vi "test_ccd_OpenAndClose.vi"(8 "error in":errorcluster, 11 "CCD in":refnum<class "CCD.lvclass">) -> (0 "error out":errorcluster, 3 "CCD out":refnum<class "CCD.lvclass">)   [LabVIEW 2020, in "horiba.test.lvlib"]
uses:
  horiba.test.lvlib
  <vilib>/addons/_JKI Toolkits/Caraya/classes/Assert/Assert True.vi
  <vilib>/addons/_JKI Toolkits/Caraya/classes/Assert/Assert False.vi
  Classes/CCD/CCD.lvclass
panel:
  # "Connector Pane"
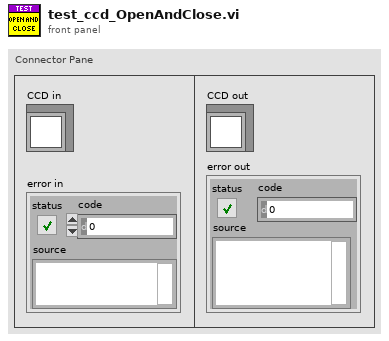
[diagram p1: front panel]
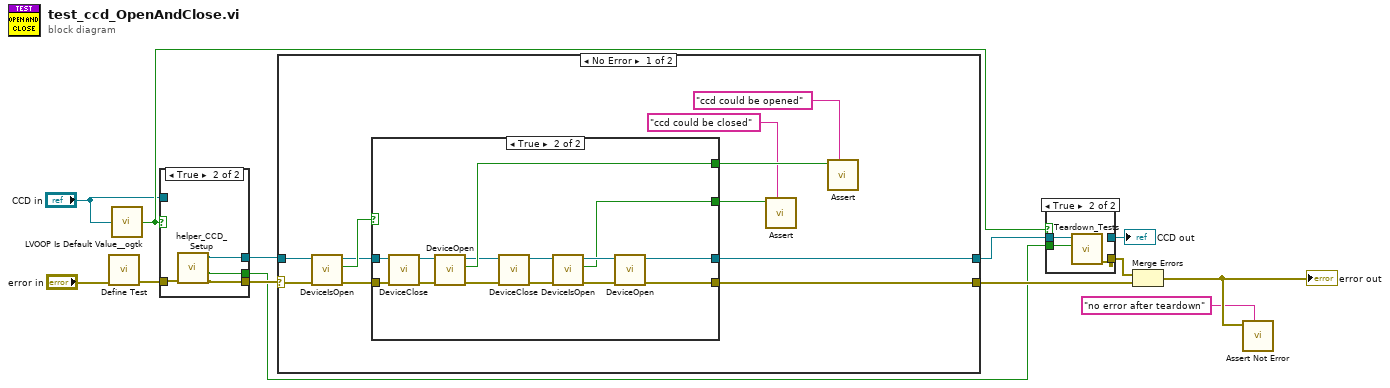
[diagram p0: block diagram]
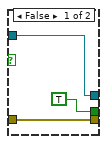
[diagram p3: hidden frame]
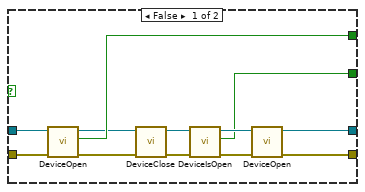
[diagram p4: hidden frame]
diagram:
  n1 = call <vilib>:"Define Test.vi"("error in (no error)"="error in") -> ("error out"=w9:errorcluster)  [unwired: 9 in, 1 out]
  n2 = call <userlib>:"LVOOP Is Default Value__ogtk.vi"("Object"="CCD in") -> ("Is Default Value?"=w3:bool)
  n3 = case shown="True" w3 {
    tunnel: w9 -> [w16 w17]
    tunnel: [w16 w19] -> w8
    tunnel: [w14 w20] -> w7
    tunnel: [TRUE ("Module Was Already Running?") w18] -> w4
    tunnel: "CCD in" -> [w14 _]
    frame False {
    }
    frame True {
      n4 = call "helper_CCD_Setup.vi"("error in"=w17) -> ("error out"=w19:errorcluster, "Module Was Already Running?"=w18:bool, "CCD out"=w20:refnum<class "CCD.lvclass">)  [unwired: 7 in, 1 out]
    }
  }
  n5 = case shown="No Error" w8 {
    selector: w8 -> [w30 w59]
    tunnel: [w21 w58] -> w12
    tunnel: w7 -> [w31 w58]
    tunnel: [w22 w59] -> w11
    frame No Error {
      n6 = call-dynamic "DeviceIsOpen.vi"("error in (no error)"=w30, "CCD in"=w31) -> ("error out"=w27:errorcluster, "device is open?"=w29:bool, "CCD out"=w28:refnum<class "CCD.lvclass">)  [unwired: 6 in, 1 out]
      n7 = case shown="True" w29 {
        tunnel: w28 -> [w42 w47]
        tunnel: w27 -> [w43 w48]
        tunnel: [w41 w57] -> w26
        tunnel: [w32 w44] -> w23
        tunnel: [w34 w50] -> w22
        tunnel: [w33 w49] -> w21
        frame False {
          n8 = call-dynamic "DeviceOpen.vi"("error in (no error)"=w43, "CCD in"=w42) -> ("error out"=w40:errorcluster, "device is open?"=w41:bool, "CCD out"=w39:refnum<class "CCD.lvclass">)  [unwired: 6 in, 1 out]
          n9 = call-dynamic "DeviceClose.vi"("error in (no error)"=w40, "CCD in"=w39) -> ("error out"=w38:errorcluster, "CCD out"=w37:refnum<class "CCD.lvclass">)  [unwired: 5 in, 3 out]
          n10 = call-dynamic "DeviceIsOpen.vi"("error in (no error)"=w38, "CCD in"=w37) -> ("error out"=w35:errorcluster, "device is open?"=w32:bool, "CCD out"=w36:refnum<class "CCD.lvclass">)  [unwired: 6 in, 1 out]
          n11 = call-dynamic "DeviceOpen.vi"("error in (no error)"=w35, "CCD in"=w36) -> ("error out"=w34:errorcluster, "CCD out"=w33:refnum<class "CCD.lvclass">)  [unwired: 6 in, 2 out]
        }
        frame True {
          n12 = call-dynamic "DeviceClose.vi"("error in (no error)"=w48, "CCD in"=w47) -> ("error out"=w45:errorcluster, "CCD out"=w46:refnum<class "CCD.lvclass">)  [unwired: 5 in, 3 out]
          n13 = call-dynamic "DeviceOpen.vi"("error in (no error)"=w45, "CCD in"=w46) -> ("error out"=w56:errorcluster, "device is open?"=w57:bool, "CCD out"=w55:refnum<class "CCD.lvclass">)  [unwired: 6 in, 1 out]
          n14 = call-dynamic "DeviceClose.vi"("error in (no error)"=w56, "CCD in"=w55) -> ("error out"=w54:errorcluster, "CCD out"=w53:refnum<class "CCD.lvclass">)  [unwired: 5 in, 3 out]
          n15 = call-dynamic "DeviceIsOpen.vi"("error in (no error)"=w54, "CCD in"=w53) -> ("error out"=w51:errorcluster, "device is open?"=w44:bool, "CCD out"=w52:refnum<class "CCD.lvclass">)  [unwired: 6 in, 1 out]
          n16 = call-dynamic "DeviceOpen.vi"("error in (no error)"=w51, "CCD in"=w52) -> ("error out"=w50:errorcluster, "CCD out"=w49:refnum<class "CCD.lvclass">)  [unwired: 6 in, 2 out]
        }
      }
      n17 = call-poly <vilib>:"Assert.vi"("Label"="ccd could be closed", "False?"=w23) -> ()  [unwired: 8 in, 2 out]
      n18 = call-poly <vilib>:"Assert.vi"("Label"="ccd could be opened", "True?"=w26) -> ()  [unwired: 8 in, 2 out]
    }
    frame Error {
    }
  }
  n19 = case shown="True" w3 {
    tunnel: w12 -> [w60 w63]
    tunnel: [_ w62] -> w6
    tunnel: w4 -> [_ w61]
    tunnel: [w60 _] -> w1
    frame False {
    }
    frame True {
      n20 = call "Teardown_Tests.vi"("Module Was Already Running?"=w61, "horiba.lvlib:GenericDevice"=w63) -> ("error out"=w62:errorcluster)  [unwired: 8 in, 1 out]
    }
  }
  "CCD out" <- w1
  n21 = Merge Errors(w6, w11) -> (w10:errorcluster)
  "error out" <- w10
  n22 = call <vilib>:"Assert Not Error.vi"("Label"="no error after teardown", "Not Error?"=w10) -> ()  [unwired: 8 in, 2 out]
